vi "Check for Throttle.vi"(8 "error in (no error)":errorcluster, 11 "Command Processor Actor in":refnum<class "Command Processor Actor.lvclass">) -> (0 "error out":errorcluster, 2 "Should Throttle":bool, 3 "Command Processor Actor out":refnum<class "Command Processor Actor.lvclass">)   [LabVIEW 2014, in "Robot Actor Framework.lvlib" / "Command Processor Actor.lvlib" / "Command Processor Actor.lvclass"]
uses:
  Command Processor Actor.lvclass
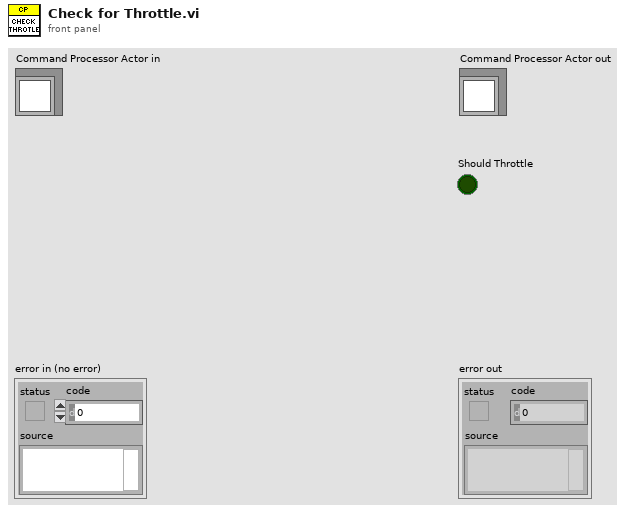
[diagram p1: front panel]
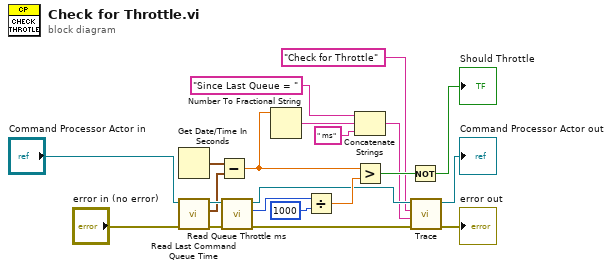
[diagram p0: block diagram]
diagram:
  n1 = Get Date/Time In Seconds() -> (seconds since 1Jan1904=w12:timestamp)
  n2 = call-dynamic "Read Last Command Queue Time.vi"("error in (no error)"="error in (no error)", "Command Processor Actor in"="Command Processor Actor in") -> ("error out"=w13:errorcluster, "Last Command Start Time"=w11:timestamp, "Command Processor Actor out"=w18:refnum<class "Command Processor Actor.lvclass">)  [unwired: 7 in]
  n3 = Subtract(x=w12, y=w11) -> (x-y=w8:dbl)
  n4 = call-dynamic "Read Queue Throttle ms.vi"("error in (no error)"=w13, "Command Processor Actor in"=w18) -> ("error out"=w2:errorcluster, "Queue Throttle ms"=w17:u32, "Command Processor Actor out"=w5:refnum<class "Command Processor Actor.lvclass">)  [unwired: 7 in]
  n5 = Number To Fractional String(number=w8) -> (F-format string=w7:string)  [unwired: 3 in]
  n6 = Divide(x=w17, y=u32 1000 ("x")) -> (x/y=w15:dbl)
  n7 = Concatenate Strings("Since Last Queue = " ("Trace Message"), w7, " ms" ("string")) -> (w4:string)
  n8 = Greater?(x=w8, y=w15) -> (0:w14:bool)
  n9 = Not(x=w14) -> (.not. x?=→"Should Throttle":bool)
  n10 = call-dynamic "Trace.vi"("error in (no error)"=w2, "Command Processor Message"=w4, "Command Processor Action"="Check for Throttle", "Command Processor Actor in"=w5) -> ("error out"=→"error out":errorcluster, "Command Processor Actor out"=→"Command Processor Actor out":refnum<class "Command Processor Actor.lvclass">)  [unwired: 6 in]
